vi "Receive Message.vi"(6 "priority":i32, 10 "Caller in":refnum<class "Caller.lvclass">, 11 "Message in":refnum<class "Message.lvclass">) -> (0 "error out":errorcluster, 2 "Actor out":refnum<class "Actor.lvclass">)   [LabVIEW 2020, in "Caller.lvlib" / "Caller.lvclass"]
doc: "This VI should be overriden ONLY if you are creating a proxy actor for remote transmission. If you are, override this VI to transmit the received message to a new destination, maintaining the given priority."
uses:
  Caller.lvclass
  <vilib>/ActorFramework/Message/Message.lvclass
  <vilib>/ActorFramework/Actor/Actor.lvclass
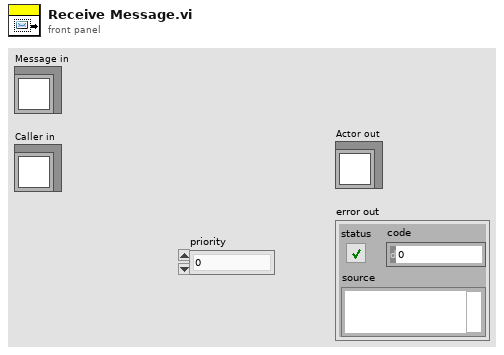
[diagram p1: front panel]
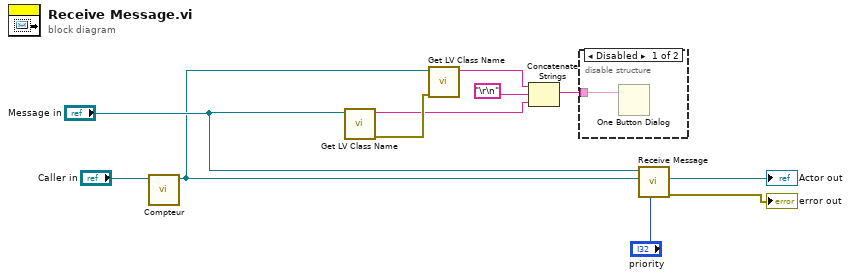
[diagram p0: block diagram]
diagram:
  n1 = call "Compteur.vi"("Caller in"="Caller in") -> ("Caller out"=w5:refnum<class "Caller.lvclass">)  [unwired: 9 in, 1 out]
  n2 = call <vilib>:"Get LV Class Name.vi"("object"="Message in") -> ("error out"=w7:errorcluster, "class name"=w3:string)  [unwired: 9 in]
  n3 = call <vilib>:"Get LV Class Name.vi"("error in (no error)"=w7, "object"=w5) -> ("class name"=w4:string)  [unwired: 8 in, 1 out]
  n4 = Concatenate Strings(w4, "\r\n", w3) -> (w1:string)
  n5 = disable-structure shown="Disabled" {
    disable-tunnel: w1 -> [w12 _]
    frame Disabled {
      n6 = One Button Dialog(message=w12) -> ()  [unwired: 1 in, 1 out]
    }
    frame Enabled {
    }
  }
  n7 = call-parent "Receive Message.vi"("priority"="priority", "Actor in"=w5, "Message in"="Message in") -> ("error out"=→"error out":errorcluster, "Actor out"=→"Actor out":refnum<class "Actor.lvclass">)  [unwired: 7 in]
